vi "To-string-array.vi"(8 "error in (no error)":errorcluster, 11 "Action in":refnum<class "Home.lvclass">) -> (0 "error out":errorcluster, 2 "Action string array":string[](array[string]), 3 "Action out":refnum<class "Home.lvclass">)   [LabVIEW 2013, in "PowderDeposition.lvlib" / "Home.lvclass"]
uses:
  Home.lvclass
  Home.lvclass/Home.ctl
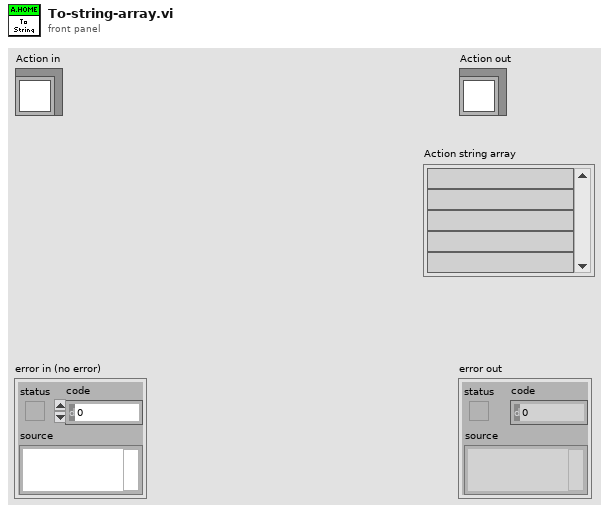
[diagram p1: front panel]
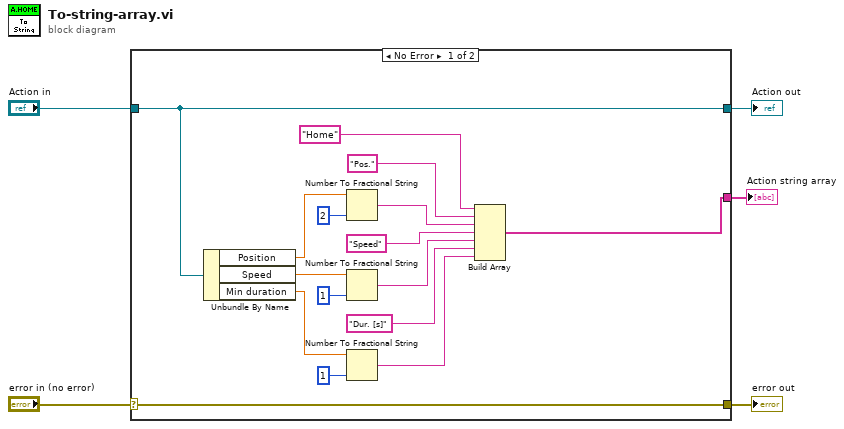
[diagram p0: block diagram]
diagram:
  n1 = case shown="No Error" "error in (no error)" {
    selector: "error in (no error)" -> [w21 w23]
    tunnel: [w21 w23] -> w4
    tunnel: [w20 w22] -> w2
    tunnel: "Action in" -> [w20 w22]
    tunnel: [w6 _] -> w1
    frame No Error {
      n2 = Unbundle By Name(w20) -> ("Position"=w19:dbl, "Speed"=w18:dbl, "Min duration"=w17:dbl)
      n3 = Number To Fractional String(number=w19, precision (6)=i16 2) -> (F-format string=w12:string)  [unwired: 2 in]
      n4 = Number To Fractional String(number=w18, precision (6)=i16 1) -> (F-format string=w10:string)  [unwired: 2 in]
      n5 = Number To Fractional String(number=w17, precision (6)=i16 1) -> (F-format string=w8:string)  [unwired: 2 in]
      n6 = Build Array("Home", "Pos.", w12, "Speed", w10, "Dur. [s]", w8) -> (w6:string[])
    }
    frame Error {
    }
  }
  "error out" <- w4
  "Action out" <- w2
  "Action string array" <- w1
